vi "Red Pitaya Current-Voltage.vi"(8 "Error In":errorcluster, 10 "Server port":u16=1002, 11 "Server address":string="192.168.1.100") -> (0 "Error Out":errorcluster)   [LabVIEW 2016]
uses:
  Mode.ctl
  Red Pitaya Parameters.ctl
  RP Command.ctl
  RP Read Temperature TCP.vi
  RP Read Status TCP.vi
  RP Write Command TCP.vi
  RP Read Subset TCP.vi
panel:
  in  "Controls":enum32{"Basic", "Advanced"}(tab)
  out "X&Y":cluster{i32, i32}(graph)
  in  "Parameters":T1={"Ranges"=[20.0, 20.0], "Output frequency 1"=15625000.0, "Output frequency 2"=50000.0, "Pre-trigger samples"=-100000, "Post-trigger samples"=11534336, "Desimation rate"=125, "Delayed start"=571428} {"Delayed start" format="0x%x (%d)"; "Post-trigger samples" format="0x%x (%d)"; "Pre-trigger samples" format="0x%x (%d)"; "Output frequency 2" format="%#_6p"; "Output frequency 1" format="%#_6p"; "Ranges" format="%#_12p"}
  out "CPU Temperature":dbl(slide)=48.847186279148 scale=0.0..100.0
  out "Y":i32=1717987 format="0x%x (%d)"
  out "X":i32=1717987 format="0x%x (%d)"
  in  "Trigger delay":u64=67108864 format="0x%x (%d)"
  in  "Read XY":bool=TRUE
  in  "Trigger pos acuracy":i32=2
  in  "Signal bits":i32=14
  in  "Read Temperature":bool=TRUE
  in  "Read trigger":bool=TRUE
  in  "Start server":bool
  in  "FPGA Logic":enum16{"Digitizer", "Fast Digitizer"}(ring)
  in  "Auto-save file":bool=TRUE
  in  "Samples to read":u64=67108864 format="0x%x (%d)"
  in  "Record":bool
  out "Server  output":string
  out "Temperature Chart":dbl(graph)=48.847186279148
  out "bytes written":i32=8
  in  "Status":bool
  out "Status response":u32=1 format="0x%x (%d)"
  out "element":u32
  in  "Status offset":u64=12
  out "Record start pos":u32=1
  out "x-y":u32=4294967295
  out "Phase increment 2":u64=1717987
  out "Phase increment 1":u64=1717987 format="0x%x (%d)"
  in  "Process Stop Button":bool
  in  "Read":bool
  in  "Read subset":bool
  out "Data File  Path":path
  out "Trigger state":bool
  in  "Trigger":bool
  in  "Arm":bool
  out "Phase  Graph":u32[](graph)
  in  "Mode":T2=enum."Digitizer"
  out "Waveform Graph":sgl[][](graph)
  in  "Stop Server":bool
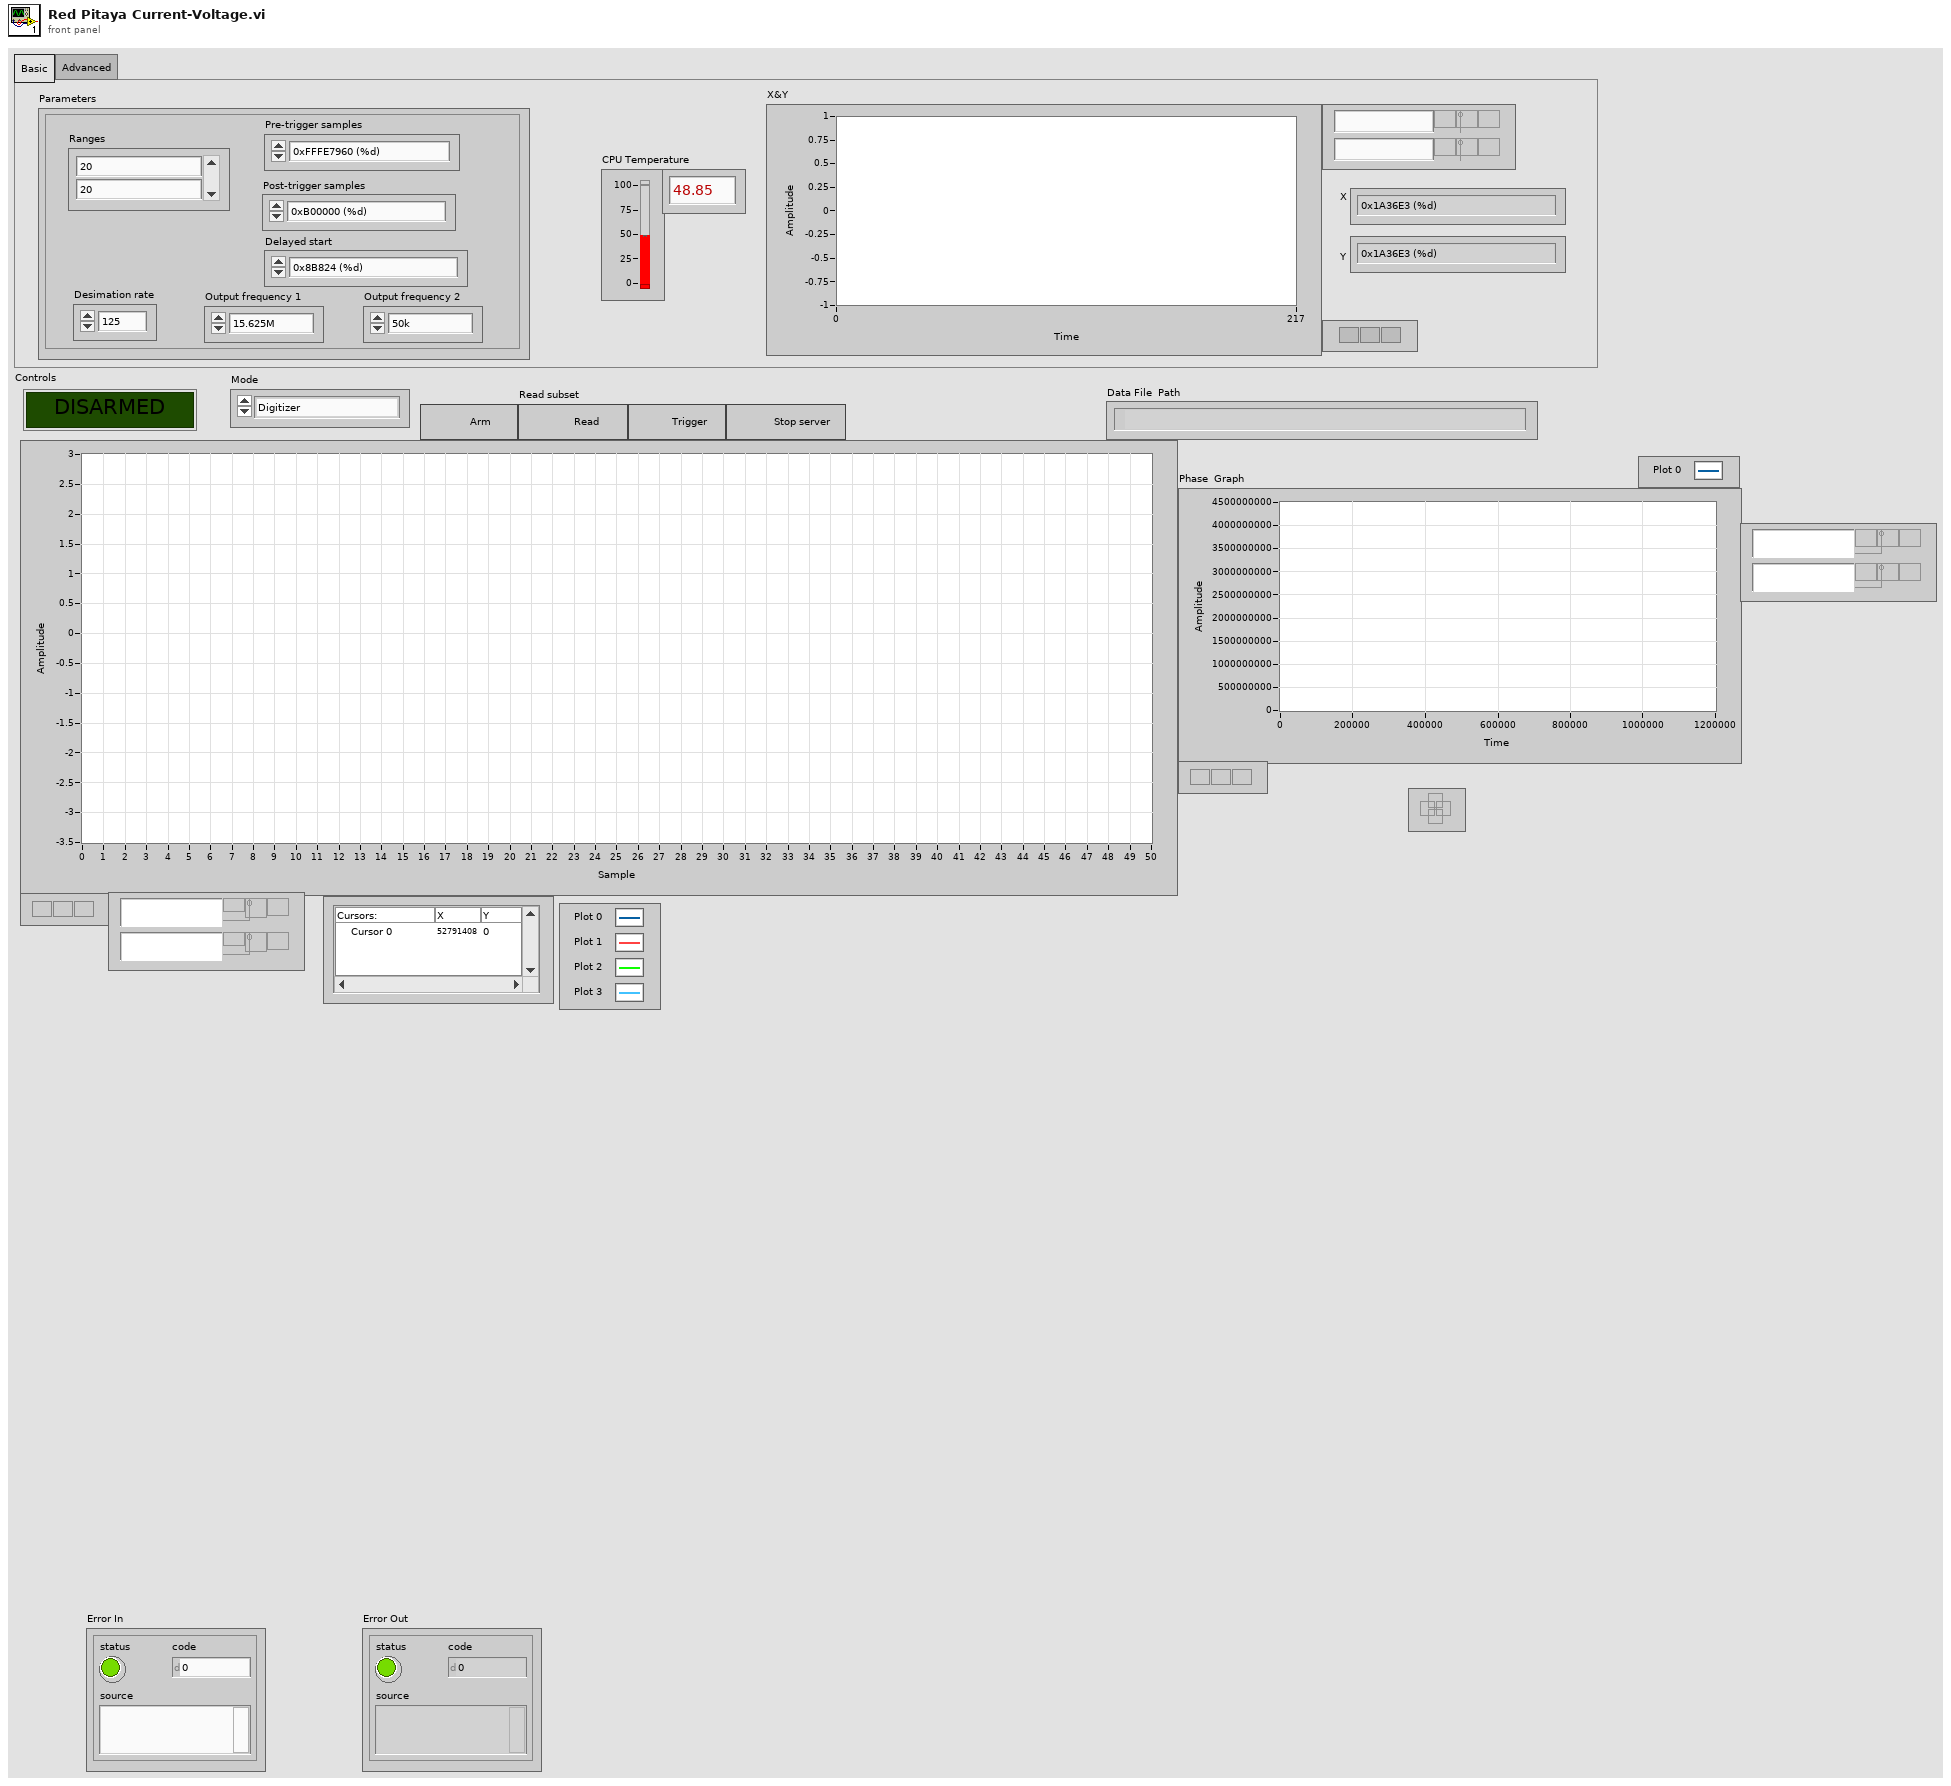
[diagram p1: front panel]
types:
  T1 = typedef "Red Pitaya Parameters.ctl" = cluster{"Ranges":dbl[], "Output frequency 1":dbl, "Output frequency 2":dbl, "Pre-trigger samples":i32, "Post-trigger samples":u64, "Desimation rate":u64, "Delayed start":u64}
  T2 = typedef "Mode.ctl" = enum16{"Filter", "Lockin test", "Snapshot test", "Digitizer", "Current-Voltage"}
  T3 = typedef "RP Command.ctl" = enum16{"Reset", "Read IDN", "Stop server", "Get status", "Get temperature", "Connect client", "Arm", "Software trigger", "Get whole buffer", "Get chunk", "System call", "Get config", "Set config", "Recieve data", "Play pattern", "Transmit data"}
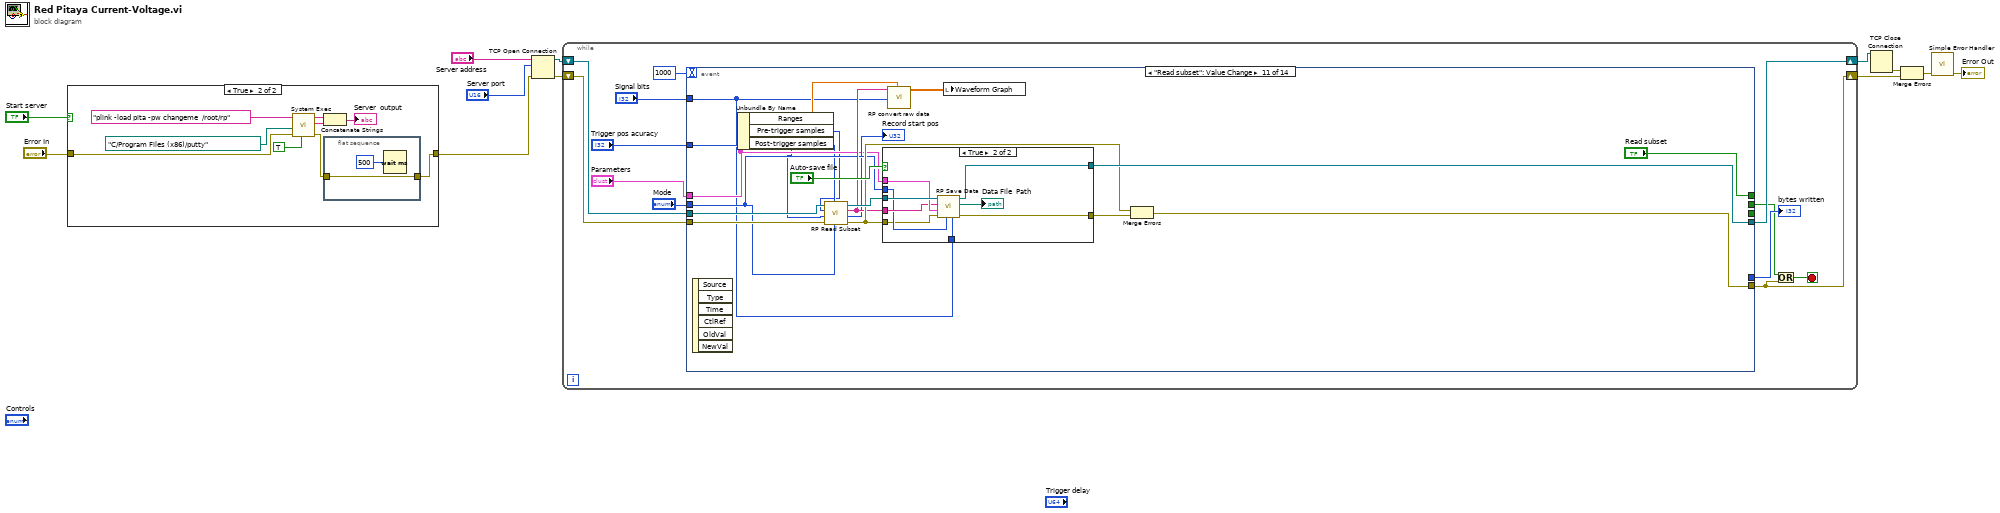
[diagram p0: block diagram]
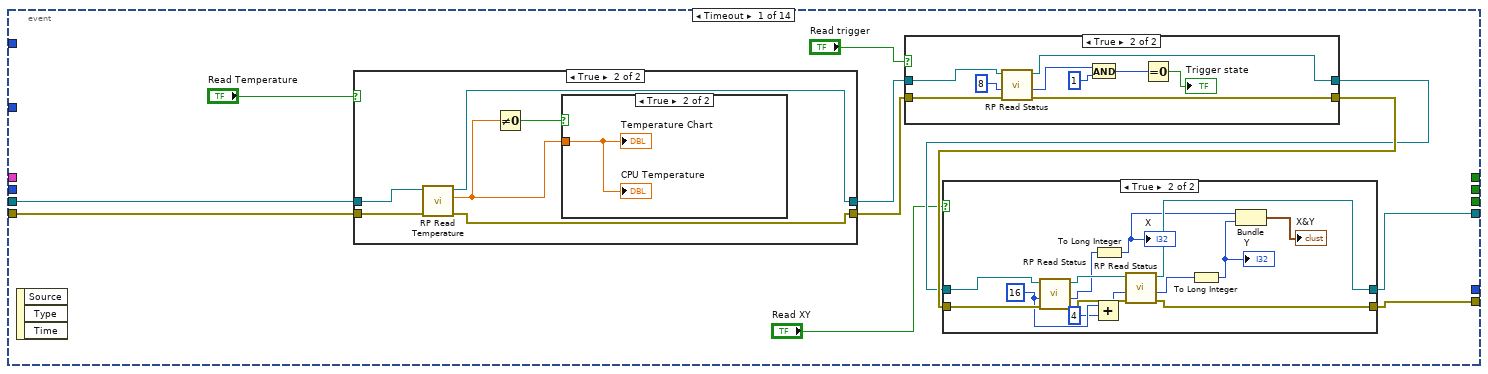
[diagram p3: hidden frame]
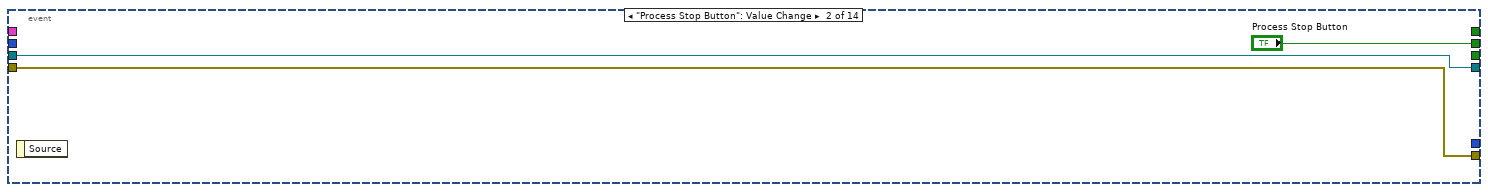
[diagram p8: hidden frame]
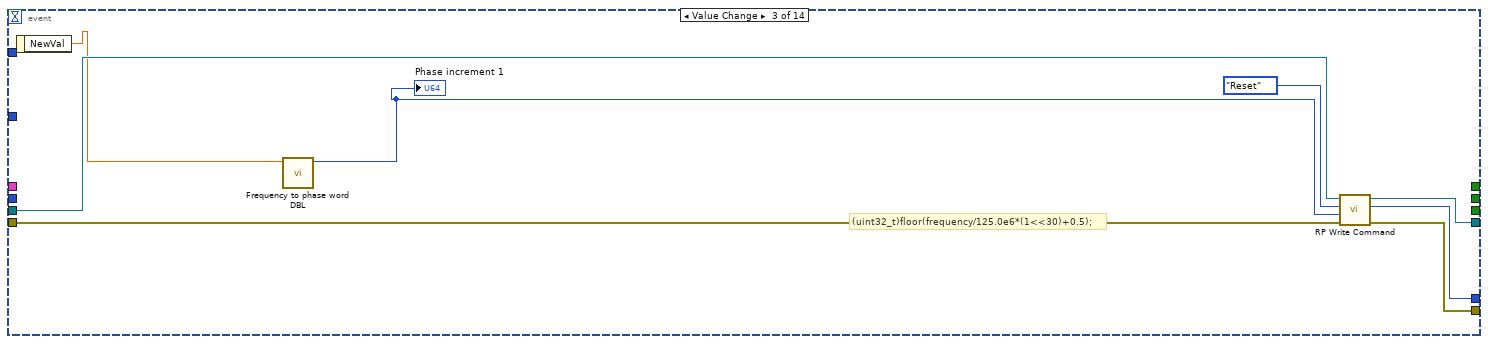
[diagram p9: hidden frame]
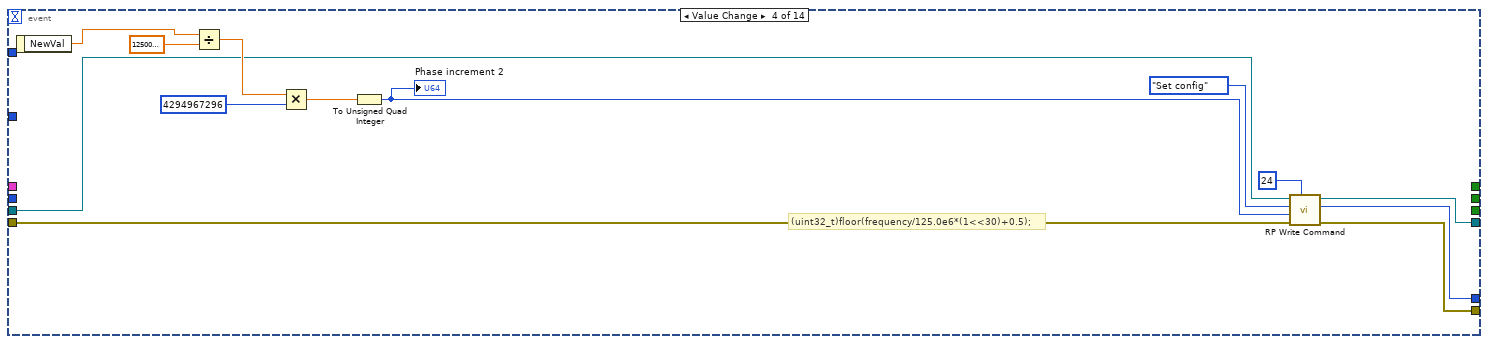
[diagram p10: hidden frame]
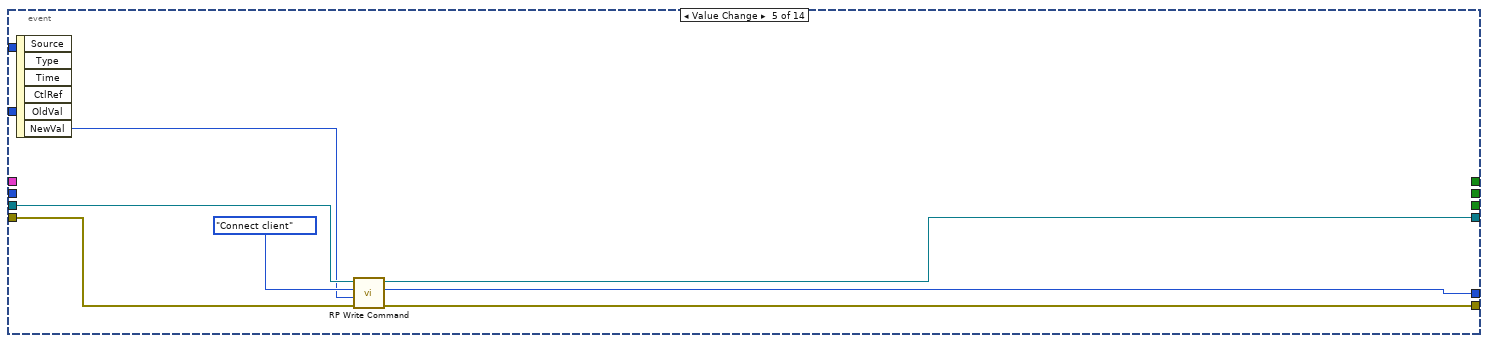
[diagram p11: hidden frame]
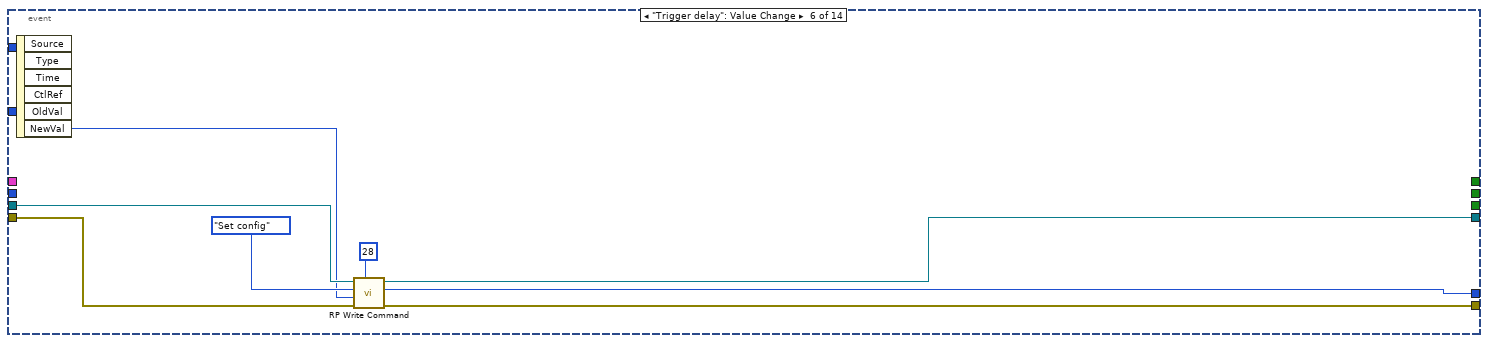
[diagram p12: hidden frame]
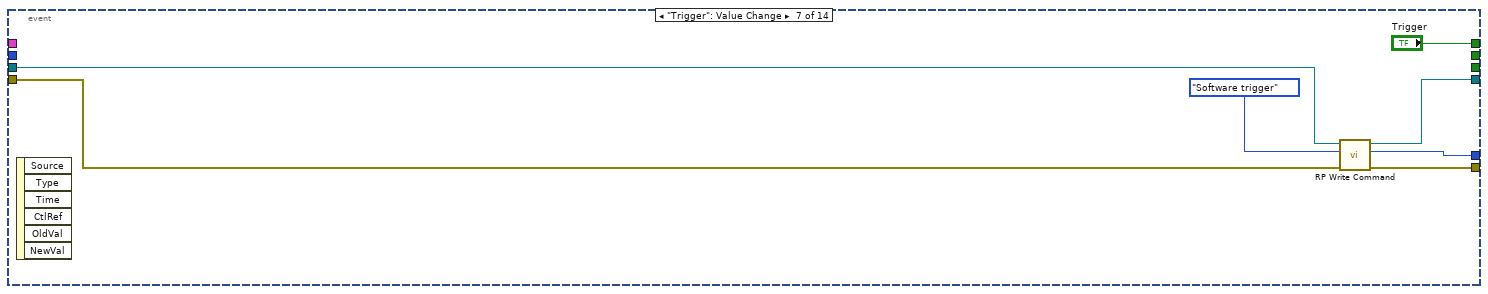
[diagram p13: hidden frame]
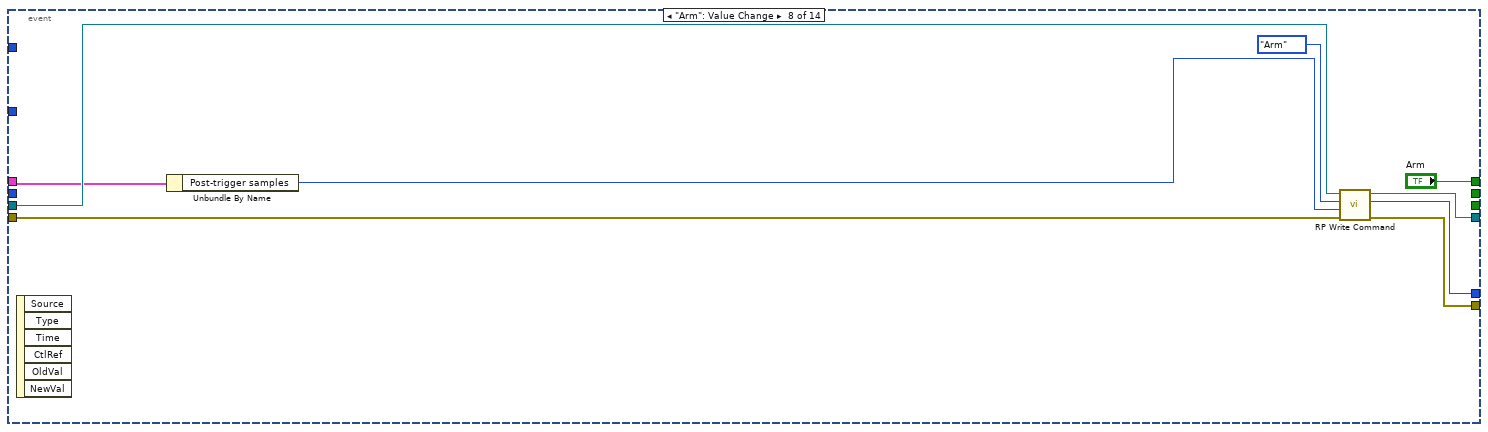
[diagram p14: hidden frame]
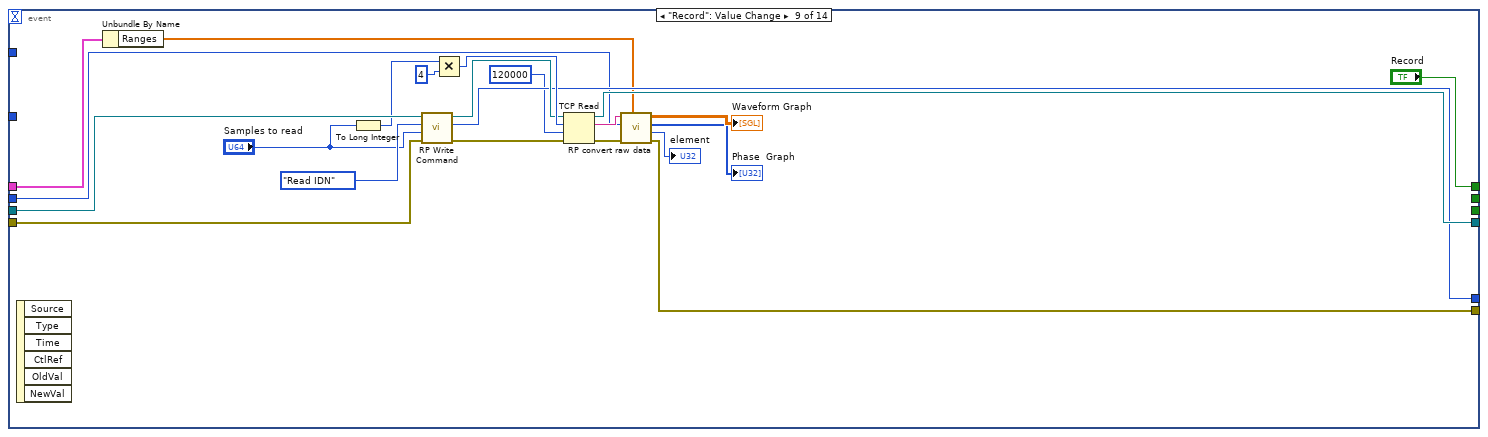
[diagram p15: hidden frame]
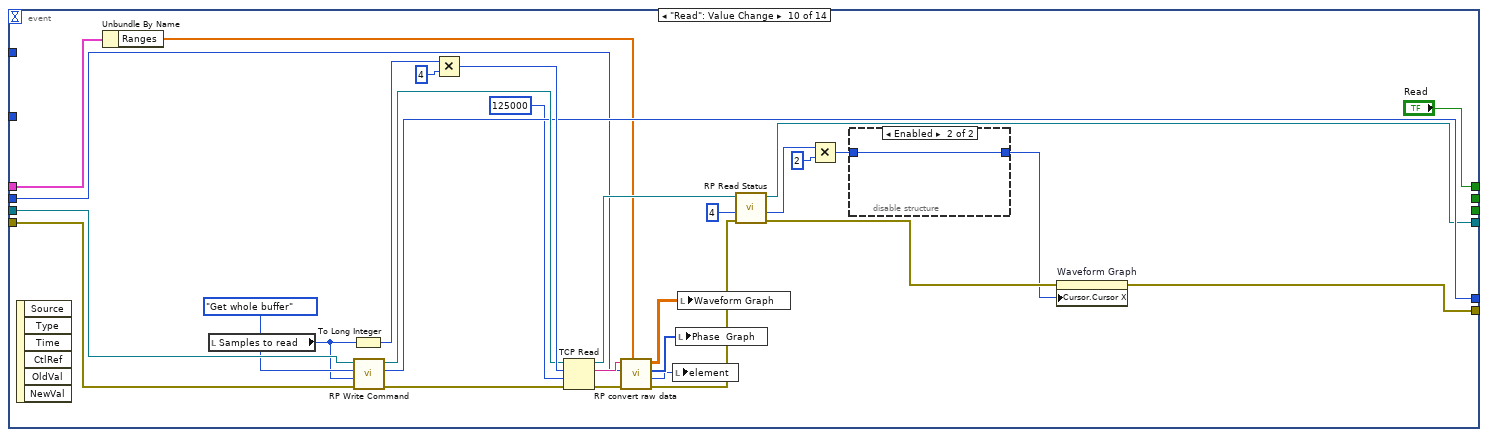
[diagram p16: hidden frame]
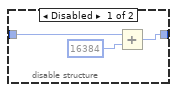
[diagram p17: hidden frame]
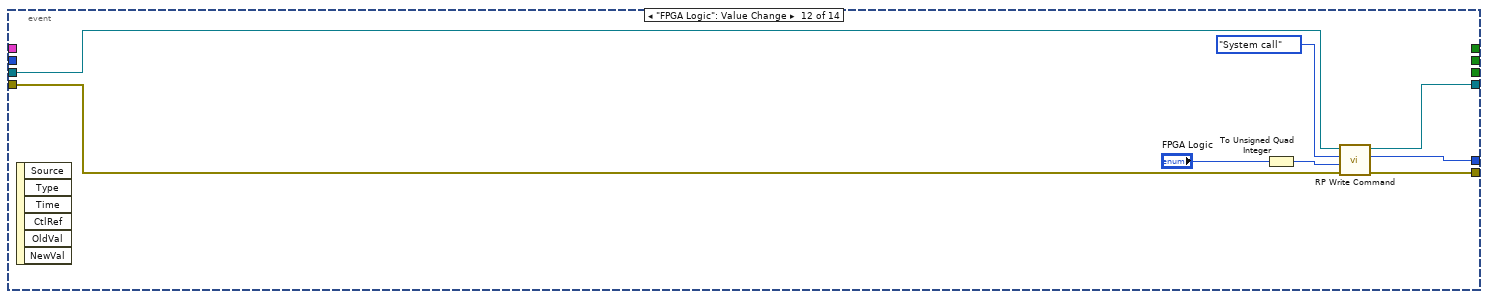
[diagram p19: hidden frame]
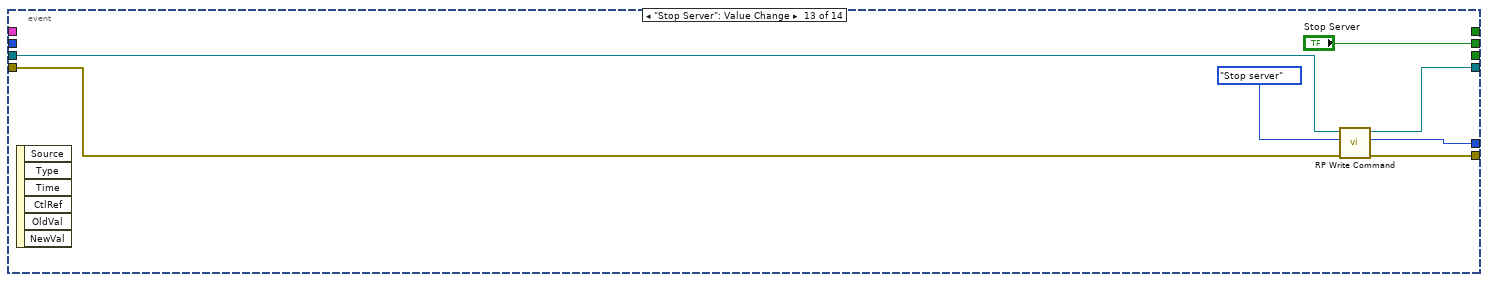
[diagram p20: hidden frame]
diagram:
  n1 = case shown="True" "Start server" {
    tunnel: [w13 w14] -> w2
    tunnel: "Error In" -> [w13 w16]
    frame False {
    }
    frame True {
      n2 = call <vilib>:"System Exec.vi"("run minimized? (F)"=TRUE, "error in (no error)"=w16, "working directory"=path "C:/Program Files (x86)/putty", "command line"="plink -load pita -pw changeme  /root/rp") -> ("error out"=w15:errorcluster, "standard error"=w18:string, "standard output"=w22:string)  [unwired: 4 in, 1 out]
      n3 = Concatenate Strings(w22, w18) -> (→"Server  output":string)
      n4 = flat-sequence {
        tunnel: w15 -> [w24]
        tunnel: [w24] -> w14
        frame #0 {
          n5 = Wait (ms)(milliseconds to wait=u32 500) -> ()  [unwired: 1 out]
        }
      }
    }
  }
  n6 = TCP Open Connection(address="Server address", remote port or service name="Server port", error in (no error)=w2) -> (connection ID=w7:refnum<k5>, error out=w8:errorcluster)  [unwired: 2 in]
  n7 = while {
    shift-right: [w34] -> w6
    shift-left: w7 -> [w35]
    shift-right: [w32] -> w5
    shift-left: w8 -> [w36]
    stop <- w30 stop-if-true
    n8 = event shown="[10] \"Read subset\": Value Change" {
      selector: _ -> [_ _ _ _ _ _ _ _ _ _ _ _ _ _]
      dyn-events: _ -> [_ _ _ _ _ _ _ _ _ _ _ _ _ _]
      timeout: 1000 -> [_ _ _ _ _ _ _ _ _ _ _ _ _ _]
      tunnel: w36 -> [w45 w85 w94 w103 w114 w122 w129 w138 w153 w185 w207 w232 w239 w245]
      tunnel: w35 -> [w46 w84 w93 w102 w113 w121 w128 w137 w156 w188 w206 w231 w237 w241]
      tunnel: [w38 w85 w90 w98 w110 w118 w125 w134 w144 w182 w211 w227 w236 w244] -> w32
      tunnel: [w39 w84 w91 w99 w111 w119 w126 w135 w158 w178 w208 w226 w235 w242] -> w34
      tunnel: [_ "Process Stop Button" _ _ _ _ _ _ _ _ _ _ "Stop Server" _] -> w31
      tunnel: [_ _ _ _ _ _ _ _ _ _ _ _ _ "Status"] -> _
      tunnel: [_ _ w89 w97 w109 w117 w124 w133 w151 w183 _ w225 w234 _] -> w33
      tunnel: [_ _ _ _ _ _ "Trigger" "Arm" "Record" "Read" "Read subset" _ _ _] -> _
      tunnel: "Mode" -> [_ _ _ _ _ _ _ _ w141 w163 w202 _ _ _]
      tunnel: "Parameters" -> [_ _ _ _ _ _ _ w131 w140 w162 w200 _ _ _]
      tunnel: "Signal bits" -> [_ _ _ _ _ _ _ _ _ _ w197 _ _ _]
      tunnel: "Trigger pos acuracy" -> [_ _ _ _ _ _ _ _ _ _ w198 _ _ _]
      event Timeout {
        n9 = event-data() -> ()  [unwired: 1 in, 3 out]
        n10 = case shown="True" "Read Temperature" {
          tunnel: w46 -> [w76 w81]
          tunnel: w45 -> [w75 w77]
          tunnel: [w76 w80] -> w43
          tunnel: [w75 w78] -> w42
          frame False {
          }
          frame True {
            n11 = call-poly "RP Read Temperature.vi"("Error In"=w77, "connection ID"=w81) -> ("error out"=w78:errorcluster, "Thermometer"=w79:dbl, "connection ID out"=w80:refnum<k5>)  [unwired: 7 in]
            n12 = Not Equal To 0?(x=w79) -> (x != 0?=w82:bool)
            n13 = case shown="True" w82 {
              tunnel: w79 -> [_ w83]
              frame False {
              }
              frame True {
                "CPU Temperature" <- w83
                "Temperature Chart" <- w83
              }
            }
          }
        }
        n14 = case shown="True" "Read trigger" {
          tunnel: w43 -> [w64 w73]
          tunnel: w42 -> [w65 w74]
          tunnel: [w65 w69] -> w41
          tunnel: [w64 w66] -> w40
          frame False {
          }
          frame True {
            n15 = call-poly "RP Read Status.vi"("Error In"=w74, "Status offset"=u64 8, "connection ID"=w73) -> ("Error Out"=w69:errorcluster, "Status response"=w71:u32, "connection ID out"=w66:refnum<k5>)  [unwired: 6 in]
            n16 = And(x=w71, y=u32 1) -> (x .and. y?=w68:u32)
            n17 = Equal To 0?(x=w68) -> (x = 0?=→"Trigger state":bool)
          }
        }
        n18 = case shown="True" "Read XY" {
          tunnel: w40 -> [w48 w62]
          tunnel: w41 -> [w49 w63]
          tunnel: [w49 w60] -> w38
          tunnel: [w48 w58] -> w39
          frame False {
          }
          frame True {
            w57 = u64 16 ("Status offset")
            n19 = call-poly "RP Read Status.vi"("Error In"=w63, "Status offset"=w57, "connection ID"=w62) -> ("Error Out"=w61:errorcluster, "Status response"=w54:u32, "connection ID out"=w59:refnum<k5>)  [unwired: 6 in]
            n20 = Add(x=w57, y=u64 4) -> (x+y=w55:u64)
            n21 = To Long Integer(number=w54) -> (32bit integer=w52:i32)
            "X" <- w52
            n22 = call-poly "RP Read Status.vi"("Error In"=w61, "Status offset"=w55, "connection ID"=w59) -> ("Error Out"=w60:errorcluster, "Status response"=w53:u32, "connection ID out"=w58:refnum<k5>)  [unwired: 6 in]
            n23 = To Long Integer(number=w53) -> (32bit integer=w51:i32)
            "Y" <- w51
            n24 = Bundle(w52, w51) -> (→"X&Y":cluster{i32, i32})  [unwired: 1 in]
          }
        }
      }
      event "Process Stop Button": Value Change {
        n25 = event-data() -> ()  [unwired: 1 in, 1 out]
      }
      event Value Change {
        # "(uint32_t)floor(frequency/125.0e6*(1<<30)+0.5);"
        n26 = event-data() -> ("NewVal"=w88:dbl)  [unwired: 1 in]
        n27 = call "Frequency to phase word DBL.vi"("Frequency"=w88) -> ("Phase word"=w87:u64)  [unwired: 10 in]
        "Phase increment 1" <- w87
        n28 = call-poly "RP Write Command.vi"("Error In"=w94, "Command payload"=w87, "Command number"=RP_Command."Reset", "connection ID"=w93) -> ("Error Out"=w90:errorcluster, "bytes written"=w89:i32, "connection ID out"=w91:refnum<k5>)  [unwired: 5 in]
      }
      event Value Change {
        # "(uint32_t)floor(frequency/125.0e6*(1<<30)+0.5);"
        n29 = event-data() -> ("NewVal"=w95:dbl)  [unwired: 1 in]
        n30 = Divide(x=w95, y=125000000.0) -> (x/y=w105:dbl)
        n31 = Multiply(x=w105, y=i64 4294967296) -> (x*y=w104:dbl)
        n32 = To Unsigned Quad Integer(1:w104) -> (0:w100:u64)
        "Phase increment 2" <- w100
        n33 = call-poly "RP Write Command.vi"("Config offset"=u64 24, "Error In"=w103, "Command payload"=w100, "Command number"=RP_Command."Set config", "connection ID"=w102) -> ("Error Out"=w98:errorcluster, "bytes written"=w97:i32, "connection ID out"=w99:refnum<k5>)  [unwired: 4 in]
      }
      event Value Change {
        n34 = event-data() -> ("NewVal"=w108:u64)  [unwired: 1 in, 5 out]
        n35 = call-poly "RP Write Command.vi"("Error In"=w114, "Command payload"=w108, "Command number"=RP_Command."Connect client", "connection ID"=w113) -> ("Error Out"=w110:errorcluster, "bytes written"=w109:i32, "connection ID out"=w111:refnum<k5>)  [unwired: 5 in]
      }
      event "Trigger delay": Value Change {
        n36 = event-data() -> ("NewVal"=w116:u64)  [unwired: 1 in, 5 out]
        n37 = call-poly "RP Write Command.vi"("Config offset"=u64 28, "Error In"=w122, "Command payload"=w116, "Command number"=RP_Command."Set config", "connection ID"=w121) -> ("Error Out"=w118:errorcluster, "bytes written"=w117:i32, "connection ID out"=w119:refnum<k5>)  [unwired: 4 in]
      }
      event "Trigger": Value Change {
        n38 = event-data() -> ()  [unwired: 1 in, 6 out]
        n39 = call-poly "RP Write Command.vi"("Error In"=w129, "Command number"=RP_Command."Software trigger", "connection ID"=w128) -> ("Error Out"=w125:errorcluster, "bytes written"=w124:i32, "connection ID out"=w126:refnum<k5>)  [unwired: 6 in]
      }
      event "Arm": Value Change {
        n40 = event-data() -> ()  [unwired: 1 in, 6 out]
        n41 = Unbundle By Name(w131) -> ("Post-trigger samples"=w130:u64)
        n42 = call-poly "RP Write Command.vi"("Error In"=w138, "Command payload"=w130, "Command number"=RP_Command."Arm", "connection ID"=w137) -> ("Error Out"=w134:errorcluster, "bytes written"=w133:i32, "connection ID out"=w135:refnum<k5>)  [unwired: 5 in]
      }
      event "Record": Value Change {
        n43 = event-data() -> ()  [unwired: 1 in, 6 out]
        n44 = Unbundle By Name(w140) -> ("Ranges"=w139:dbl[])
        n45 = To Long Integer(number="Samples to read") -> (32bit integer=w150:i32)
        n46 = call-poly "RP Write Command.vi"("Error In"=w153, "Command payload"="Samples to read", "Command number"=RP_Command."Read IDN", "connection ID"=w156) -> ("Error Out"=w152:errorcluster, "bytes written"=w151:i32, "connection ID out"=w154:refnum<k5>)  [unwired: 5 in]
        n47 = Multiply(x=w150, y=4) -> (x*y=w157:i32)
        n48 = TCP Read(connection ID=w154, bytes to read=w157, error in (no error)=w152, 9:120000 ("timeout ms (25000)")) -> (connection ID out=w158:refnum<k5>, data out=w147:string, error out=w145:errorcluster)  [unwired: 1 in]
        n49 = call "RP convert raw data.vi"("Max Volts"=w139, "Error In"=w145, "Format"=w141, "data stream"=w147) -> ("Error Out"=w144:errorcluster, "element"=→"element":u32, "phase out"=→"Phase  Graph":u32[], "data out"=→"Waveform Graph":sgl[][])  [unwired: 4 in]
      }
      event "Read": Value Change {
        n50 = event-data() -> ()  [unwired: 1 in, 6 out]
        n51 = Unbundle By Name(w162) -> ("Ranges"=w161:dbl[])
        n52 = local read "Samples to read"() -> (w177:u64)
        n53 = To Long Integer(number=w177) -> (32bit integer=w180:i32)
        n54 = call-poly "RP Write Command.vi"("Error In"=w185, "Command payload"=w177, "Command number"=RP_Command."Get whole buffer", "connection ID"=w188) -> ("Error Out"=w184:errorcluster, "bytes written"=w183:i32, "connection ID out"=w186:refnum<k5>)  [unwired: 5 in]
        n55 = Multiply(x=w180, y=4) -> (x*y=w189:i32)
        n56 = TCP Read(connection ID=w186, bytes to read=w189, error in (no error)=w184, 9:125000 ("timeout ms (25000)")) -> (connection ID out=w179:refnum<k5>, data out=w175:string, error out=w165:errorcluster)  [unwired: 1 in]
        n57 = call "RP convert raw data.vi"("Max Volts"=w161, "Error In"=w165, "Format"=w163, "data stream"=w175) -> ("Error Out"=w164:errorcluster, "element"=w172:u32, "phase out"=w173:u32[], "data out"=w174:sgl[][])  [unwired: 4 in]
        n58 = local write "element"(w172) -> ()
        n59 = local write "Phase  Graph"(w173) -> ()
        n60 = local write "Waveform Graph"(w174) -> ()
        n61 = call-poly "RP Read Status.vi"("Error In"=w164, "Status offset"=u64 4, "connection ID"=w179) -> ("Error Out"=w170:errorcluster, "Status response"=w169:u32, "connection ID out"=w178:refnum<k5>)  [unwired: 6 in]
        n62 = Multiply(x=w169, y=u32 2) -> (x*y=w167:u32)
        n63 = disable-structure shown="Enabled" {
          disable-tunnel: w167 -> [w193 w194]
          disable-tunnel: [w191 w194] -> w166
          frame Disabled {
            n64 = Add(x=w193, y=16384) -> (x+y=w191:u32)
          }
          frame Enabled {
          }
        }
        n65 = property on="Waveform Graph" class="WFGraph (strict)"(error in=w170, "Cursor.Cursor X"=w166) -> (error out=w182:errorcluster)  [unwired: 1 in, 1 out]
      }
      event "Read subset": Value Change {
        n66 = event-data() -> ()  [unwired: 1 in, 6 out]
        n67 = Unbundle By Name(w200) -> ("Ranges"=w199:dbl[], "Pre-trigger samples"=w196:i32, "Post-trigger samples"=w195:u64)
        n68 = call-poly "RP Read Subset.vi"("Bytes per sample"=w202, "Samples per trigger increment"=w198, "Error In"=w207, "Post-trigger samples"=w195, "Pre-trigger samples"=w196, "connection ID"=w206) -> ("Error Out"=w204:errorcluster, "Record start pos"=→"Record start pos":u32, "Data stream"=w203:string, "connection ID out"=w205:refnum<k5>)  [unwired: 2 in]
        n69 = case shown="True" "Auto-save file" {
          tunnel: w204 -> [w215 w218]
          tunnel: w203 -> [_ w222]
          tunnel: [w215 w217] -> w210
          tunnel: w205 -> [w214 w224]
          tunnel: [w214 w220] -> w208
          tunnel: w200 -> [_ w223]
          tunnel: w202 -> [_ w221]
          tunnel: w197 -> [_ w216]
          frame False {
          }
          frame True {
            n70 = call "RP Save Data.vi"("Signal bits"=w216, "Mode"=w221, "Error In"=w218, "Parameters"=w223, "Data stream"=w222, "connection ID"=w224) -> ("Error Out"=w217:errorcluster, "Data File  Path"=→"Data File  Path":path, "connection ID out"=w220:refnum<k5>)  [unwired: 2 in, 1 out]
          }
        }
        n71 = call "RP convert raw data.vi"("Max Volts"=w199, "Signal bits"=w197, "data stream"=w203) -> ("data out"=w209:sgl[][])  [unwired: 5 in, 3 out]
        n72 = local write "Waveform Graph"(w209) -> ()
        n73 = Merge Errors(w204, w210) -> (w211:errorcluster)
      }
      event "FPGA Logic": Value Change {
        n74 = event-data() -> ()  [unwired: 1 in, 6 out]
        n75 = To Unsigned Quad Integer(1:"FPGA Logic") -> (0:w229:u64)
        n76 = call-poly "RP Write Command.vi"("Error In"=w232, "Command payload"=w229, "Command number"=RP_Command."System call", "connection ID"=w231) -> ("Error Out"=w227:errorcluster, "bytes written"=w225:i32, "connection ID out"=w226:refnum<k5>)  [unwired: 5 in]
      }
      event "Stop Server": Value Change {
        n77 = event-data() -> ()  [unwired: 1 in, 6 out]
        n78 = call-poly "RP Write Command.vi"("Error In"=w239, "Command number"=RP_Command."Stop server", "connection ID"=w237) -> ("Error Out"=w236:errorcluster, "bytes written"=w234:i32, "connection ID out"=w235:refnum<k5>)  [unwired: 6 in]
      }
      event "Status": Value Change {
        (unwired) u64 12 ("Status offset")
        n79 = event-data() -> ()  [unwired: 1 in, 6 out]
        n80 = local read "element"() -> (w247:u32)
        n81 = call-poly "RP Read Status.vi"("Error In"=w245, "Status offset"="Status offset", "connection ID"=w241) -> ("Error Out"=w244:errorcluster, "Status response"=w243:u32, "connection ID out"=w242:refnum<k5>)  [unwired: 6 in]
        "Status response" <- w243
        n82 = Subtract(x=w247, y=w243) -> (x-y=→"x-y":u32)
      }
    }
    "bytes written" <- w33
    n83 = Or(x=w31, y=w32) -> (x .or. y?=w30:bool)
  }
  n84 = TCP Close Connection(connection ID=w6) -> (error out=w10:errorcluster)  [unwired: 2 in, 1 out]
  n85 = Merge Errors(w10, w5) -> (w9:errorcluster)
  n86 = call <vilib>:"Simple Error Handler.vi"("error in (no error)"=w9) -> ("error out"=→"Error Out":errorcluster)  [unwired: 4 in, 4 out]
